vi "wavecal.vi"() -> ()   [LabVIEW 2014]
panel:
  out "port 2":u16
  out "address":u32
  in  "stop":bool
  out "boolean pin 7":bool
  in  "flipper (pin 7)":bool
  out "data out":string
  out "return String length":i32
  out "Boolean 5":bool
  out "Boolean 4":bool
  out "Boolean 3":bool
  out "Boolean 2":bool
  out "Boolean":bool
  in  "1310nm":bool
  in  "1120nm":bool
  in  "980nm":bool
  in  "920nm":bool
  in  "808nm":bool
  out "error out":errorcluster
  out "port":u16
  # "off = pupil plane\non = focal plane"
  # "changed 904nm to\n920nm on 20170924"
  # "C:\\Users\\kids\\Documents\\Arduino\\wavecal\\wavecal.ino"
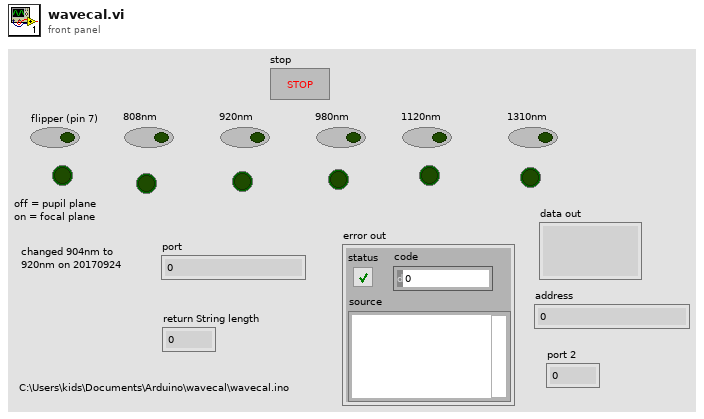
[diagram p1: front panel]
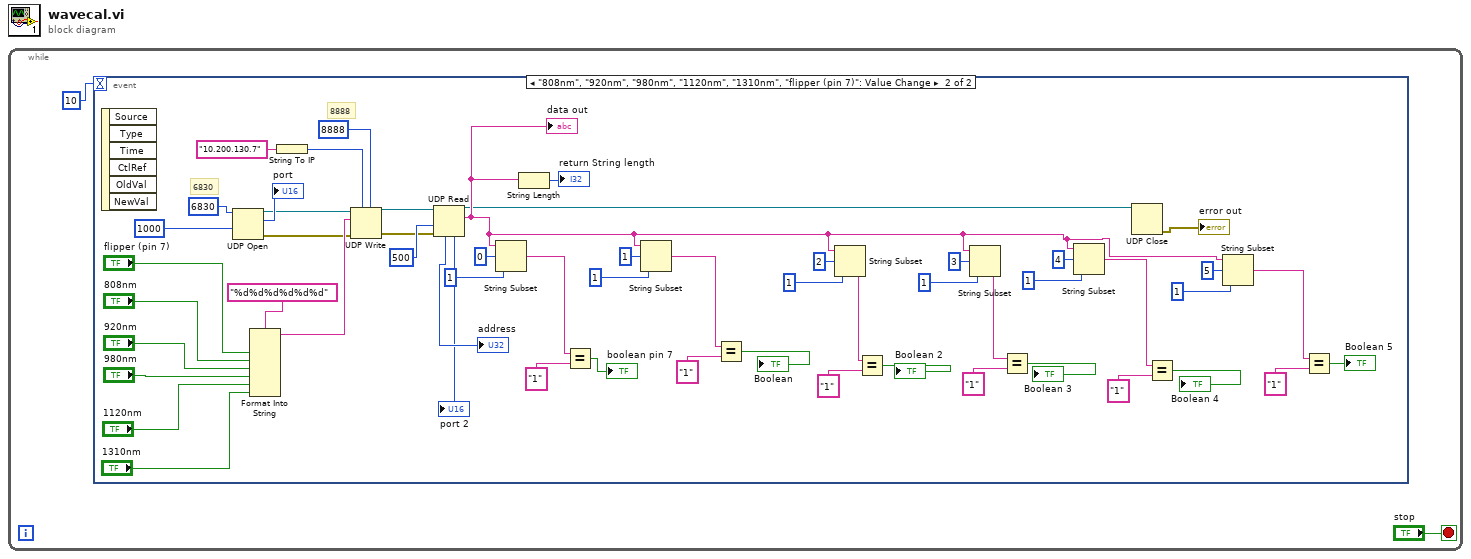
[diagram p0: block diagram]
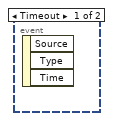
[diagram p2: hidden frame]
diagram:
  n1 = while {
    stop <- "stop" stop-if-true
    n2 = event shown="[1] \"808nm\", \"920nm\", \"980nm\", \"1120nm\", \"1310nm\", \"flipper (pin 7)\": Value Change" {
      selector: _ -> [_ _]
      dyn-events: _ -> [_ _]
      timeout: 10 -> [_ _]
      event Timeout {
        n3 = event-data() -> ()  [unwired: 1 in, 3 out]
      }
      event "808nm", "920nm", "980nm", "1120nm", "1310nm", "flipper (pin 7)": Value Change {
        # "6830"
        # "8888"
        n4 = event-data() -> ()  [unwired: 1 in, 6 out]
        n5 = UDP Open(9:1000 ("timeout ms (25000)"), 11:u16 6830 ("port")) -> (port=w7:refnum<k16>, 0:w8:errorcluster, 2:→"port":u16)  [unwired: 3 in]
        n6 = Format Into String(format string="%d%d%d%d%d%d", "flipper (pin 7)", "808nm", "920nm", "980nm", "1120nm", "1310nm") -> (resulting string=w21:string)  [unwired: 2 in, 1 out]
        n7 = String To IP(1:"10.200.130.7" ("name")) -> (0:w10:u32)
        n8 = UDP Write(address=w10, port or service name=u16 8888, connection ID=w7, data in=w21, 8:w8) -> (error out=w12:errorcluster, 3:w11:refnum<k16>)  [unwired: 1 in]
        n9 = UDP Read(connection ID=w11, timeout ms (25000)=500, 8:w12) -> (data out=w52:string, 3:w27:refnum<k16>, 4:→"port 2":u16, 6:→"address":u32)  [unwired: 1 in, 1 out]
        "data out" <- w52
        n10 = String Subset(string=w52, offset (0)=0, length (rest)=1 ("length (rest)")) -> (substring=w41:string)
        n11 = String Length(string=w52) -> (length=→"return String length":i32)
        n12 = Equal?(x=w41, y="1" ("format string")) -> (x = y?=→"boolean pin 7":bool)
        n13 = String Subset(string=w52, offset (0)=1, length (rest)=1 ("length (rest)")) -> (substring=w53:string)
        n14 = Equal?(x=w53, y="1" ("format string")) -> (x = y?=→"Boolean":bool)
        n15 = String Subset(string=w52, offset (0)=2, length (rest)=1 ("length (rest)")) -> (substring=w54:string)
        n16 = Equal?(x=w54, y="1" ("format string")) -> (x = y?=→"Boolean 2":bool)
        n17 = String Subset(string=w52, offset (0)=3, length (rest)=1 ("length (rest)")) -> (substring=w55:string)
        n18 = Equal?(x=w55, y="1" ("format string")) -> (x = y?=→"Boolean 3":bool)
        n19 = String Subset(string=w52, offset (0)=4, length (rest)=1 ("length (rest)")) -> (substring=w56:string)
        n20 = UDP Close(connection ID=w27) -> (error out=→"error out":errorcluster)  [unwired: 1 in, 1 out]
        n21 = Equal?(x=w56, y="1" ("format string")) -> (x = y?=→"Boolean 4":bool)
        n22 = String Subset(string=w52, offset (0)=5, length (rest)=1 ("length (rest)")) -> (substring=w57:string)
        n23 = Equal?(x=w57, y="1" ("format string")) -> (x = y?=→"Boolean 5":bool)
      }
    }
  }
